vi "resetActiveCycleCounter.vi"(8 "error in (no error)":errorcluster, 11 "TestMonitor in":refnum<class "TestMonitor.lvclass">) -> (0 "error out":errorcluster, 2 "activeCycle":u32, 3 "TestMonitor out":refnum<class "TestMonitor.lvclass">)   [LabVIEW 2015]
uses:
  TestMonitor.lvclass
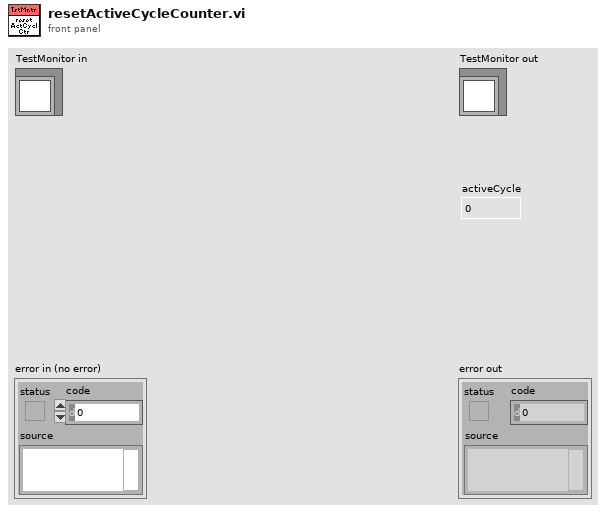
[diagram p1: front panel]
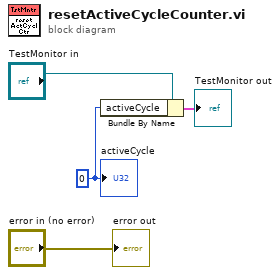
[diagram p0: block diagram]
diagram:
  w1 = u32 0 ("activeCycle")
  n1 = Bundle By Name(cluster="TestMonitor in", "activeCycle"=w1) -> (→"TestMonitor out":cluster{})
  "error out" <- "error in (no error)"
  "activeCycle" <- w1
